vi "Initialize.vi"(8 "error in":errorcluster, 10 "parameters":variant, 11 "DIO Instrument in":refnum<class "Digital IO Instrument.lvclass">) -> (0 "error out":errorcluster, 2 "summary":T2[](array[typedef]), 3 "data value reference":T1)   [LabVIEW 2025, in "Digital IO.lvlib" / "Digital IO Instrument.lvclass"]
doc: "Initializes the data of a node to its default state.\nThe object is not created inside of this VI, because it is created from a File depending on user selection.\nCopyright 2017 National Instruments Corporation\n\nLicensed under the Apache License, Version 2.0 (the \"License\"); you may not use this file except in compliance with the License. You may obtain a copy of the License at http://www.apache.org/licenses/LICENSE-2.0\nUnless required by applicable law or agreed to in writing, software distributed under the License is distributed on an \"AS IS\" BASIS, WITHOUT WARRANTIES OR CONDITIONS OF ANY KIND, either express or implied. See the License for the specific language governing permissions and limitations under the License."
uses:
  Digital IO Instrument.lvclass
  Users/Public/Documents/Sandia National Labs/TSS Plugin/CEF.lvlibp/Node/Summary.ctl
  Users/Public/Documents/Sandia National Labs/TSS Plugin/CEF.lvlibp/Node/NodeRef.ctl
  Users/Public/Documents/Sandia National Labs/TSS Plugin/CEF.lvlibp/Node/CEF_Node.lvclass
  Digital IO Instrument.lvclass/Digital IO Instrument.ctl
  Users/Public/Documents/Sandia National Labs/TSS Plugin/Abstract Engine.lvlibp/Instrument configuration/Read Instrument Setting.vi
  Users/Public/Documents/Sandia National Labs/TSS Plugin/Abstract Engine.lvlibp/Instrument configuration/Write Instrument Setting.vi
  Users/Public/Documents/Sandia National Labs/TSS Plugin/Abstract Engine.lvlibp/Abstract Instrument/Abstract Instrument.lvclass
  Users/Public/Documents/Sandia National Labs/TSS Plugin/Abstract Engine.lvlibp/Instrument configuration/Instrument configuration.lvclass
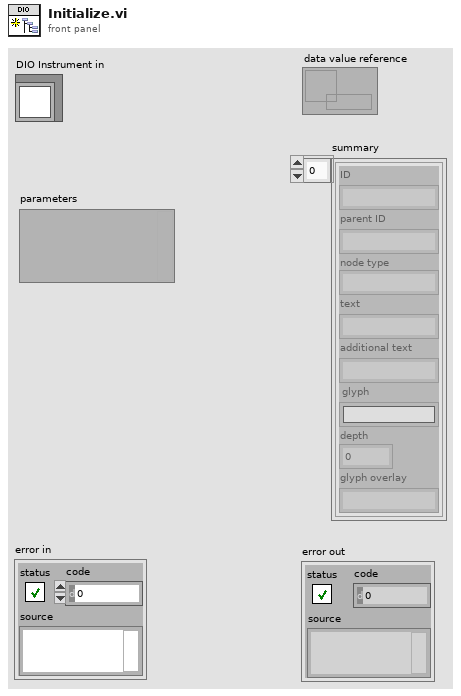
[diagram p1: front panel]
types:
  T1 = typedef "CEF.lvlibp/CEF_Node.lvclass/NodeRef.ctl" = refnum<data-value>
  T2 = typedef "CEF.lvlibp/CEF_Node.lvclass/Summary.ctl" = cluster{"ID":string, "parent ID":string, "node type":string, "text":string, "additional text":string, "glyph":string, "depth":i32, "glyph overlay":string}
  T3 = typedef "Abstract Engine.lvlibp/Instrument configuration.lvclass/Default Instrument.ctl" = cluster{"Type":string, "Address":string, "SW Alias":string, "Description":string, "Enabled":bool}
  T4 = cluster{"ID":string, "parent ID":string, "node type":string, "text":string, "additional text":string, "glyph":string, "depth":i32, "glyph overlay":string}[]
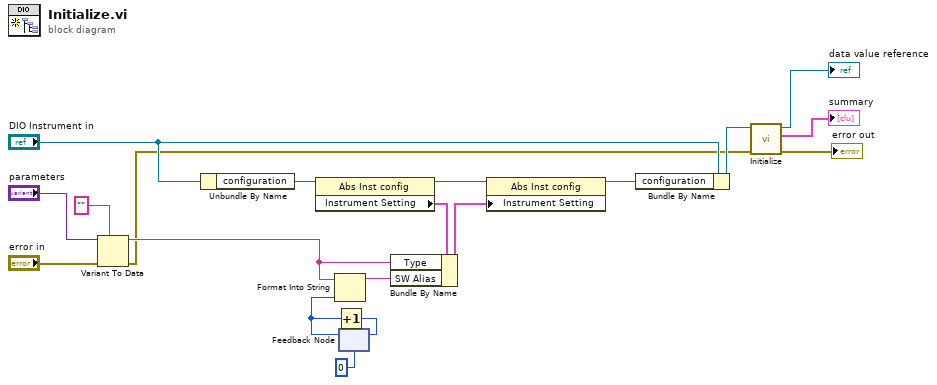
[diagram p0: block diagram]
diagram:
  n1 = Variant To Data(error in="error in", type="", Variant="parameters") -> (data=w12:string, error out=w7:errorcluster)
  n2 = Unbundle By Name("DIO Instrument in") -> ("configuration"=w6:refnum<class "Instrument configuration.lvclass">)
  n3 = property class="Abs Inst config"(reference=w6) -> (reference out=w5:refnum<class "Instrument configuration.lvclass">, "Instrument Setting"=w3:T3)  [unwired: 1 in, 1 out]
  n4 = feedback #1(0) -> (w10:i32)
  n5 = Format Into String(initial string=w12, w10) -> (resulting string=w4:string)  [unwired: 2 in, 1 out]
  n6 = Increment(x=w10) -> (x+1=w9:i32)
  n7 = feedback-in #1(w9) -> ()
  n8 = Bundle By Name(cluster=w3, "Type"=w12, "SW Alias"=w4) -> (w2:T3)
  n9 = property class="Abs Inst config"(reference=w5, "Instrument Setting"=w2) -> (reference out=w14:refnum<class "Instrument configuration.lvclass">)  [unwired: 1 in, 1 out]
  n10 = Bundle By Name(cluster="DIO Instrument in", "configuration"=w14) -> (w15:refnum<class "Digital IO Instrument.lvclass">)
  n11 = call-parent "Initialize.vi"("error in"=w7, "CEF_Serialize node in"=w15) -> ("error out"=→"error out":errorcluster, "summary"=→"summary":T4, "data value reference"=→"data value reference":refnum<data-value>)  [unwired: 7 in]
